vi "nCr_Sub_VI.vi"(10 "n 4":i32, 11 "n 3":i32) -> (3 "Numeric 2":dbl)   [LabVIEW 2024]
uses:
  <vilib>/gmath/NI_Gmath.lvlib
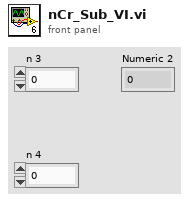
[diagram p1: front panel]
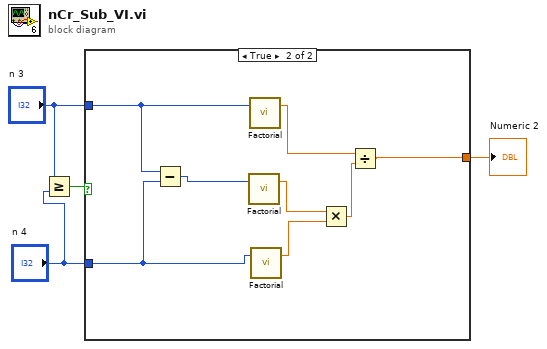
[diagram p0: block diagram]
diagram:
  n1 = Greater Or Equal?(x="n 3", y="n 4") -> (x >= y?=w1:bool)
  n2 = case shown="True" w1 {
    tunnel: "n 3" -> [_ w12]
    tunnel: "n 4" -> [_ w11]
    tunnel: [_ w5] -> w4
    frame False {
    }
    frame True {
      n3 = Subtract(x=w12, y=w11) -> (x-y=w10:i32)
      n4 = call <vilib>:"Factorial.vi"("n"=w10) -> ("n!"=w9:dbl)  [unwired: 2 in]
      n5 = call <vilib>:"Factorial.vi"("n"=w12) -> ("n!"=w7:dbl)  [unwired: 2 in]
      n6 = call <vilib>:"Factorial.vi"("n"=w11) -> ("n!"=w8:dbl)  [unwired: 2 in]
      n7 = Multiply(x=w9, y=w8) -> (x*y=w6:dbl)
      n8 = Divide(x=w7, y=w6) -> (x/y=w5:dbl)
    }
  }
  "Numeric 2" <- w4
